vi "AddPeerNodeAtIndex.vi"(8 "error in":errorcluster, 9 "TreeIndex":i32, 10 "parent node ID":string, 11 "node in":refnum<class "NISE_CEF_Node.lvclass">) -> (0 "error out":errorcluster, 2 "summary":T1[](array[typedef]))   [LabVIEW 2015, in "Configuration Tool.lvlib"]
doc: "This Vi adds a new node to the Parent Node IDCopyright 2017 National Instruments Corporation\n\nLicensed under the Apache License, Version 2.0 (the \"License\"); you may not use this file except in compliance with the License. You may obtain a copy of the License at http://www.apache.org/licenses/LICENSE-2.0\nUnless required by applicable law or agreed to in writing, software distributed under the License is distributed on an \"AS IS\" BASIS, WITHOUT WARRANTIES OR CONDITIONS OF ANY KIND, either express or implied. See the License for the specific language governing permissions and limitations under the License."
uses:
  Configuration Tool.lvlib
  <vilib>/NI/Configuration Framework/Node/Summary.ctl
  <vilib>/NI/Configuration Framework/Node/NISE_CEF_Node.lvclass
  <vilib>/NI/Configuration Framework/Node/NISE_CEF_Node.lvclass/NISE_CEF_Node.ctl
  <vilib>/NI/Configuration Framework/Node/WriteParent.vi
  <vilib>/NI/Configuration Framework/NISE_CEF_TreeControl.lvlib
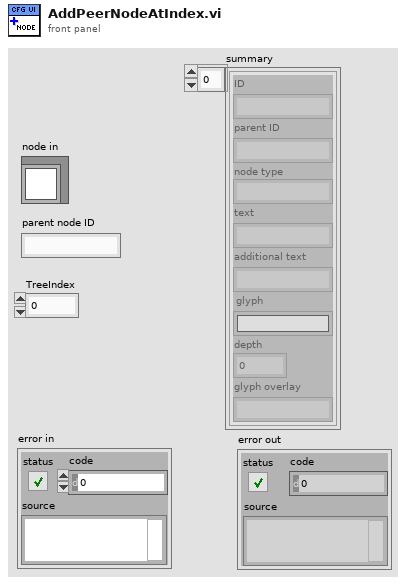
[diagram p1: front panel]
types:
  T1 = typedef "NISE_CEF_Node.lvclass/Summary.ctl" = cluster{"ID":string, "parent ID":string, "node type":string, "text":string, "additional text":string, "glyph":string, "depth":i32, "glyph overlay":string}
  T2 = typedef "NISE_CEF_Node.lvclass/NodeRef.ctl" = refnum<data-value>
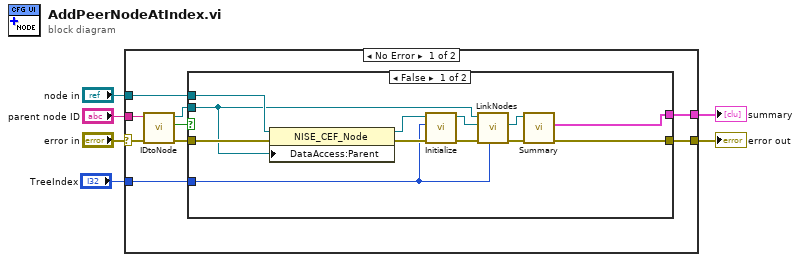
[diagram p0: block diagram]
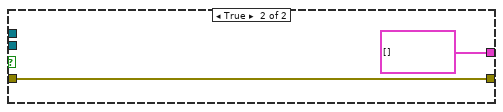
[diagram p2: hidden frame]
diagram:
  n1 = case shown="No Error" "error in" {
    selector: "error in" -> [w10 w30]
    tunnel: "parent node ID" -> [w15 _]
    tunnel: [w13 _] -> w4
    tunnel: [w12 w30] -> w3
    tunnel: "node in" -> [w11 _]
    tunnel: "TreeIndex" -> [w7 _]
    frame No Error {
      n2 = call <vilib>:"IDtoNode.vi"("error in"=w10, "ID"=w15) -> ("error out"=w9:errorcluster, "invalid Id"=w8:bool, "node ref"=w14:T2)  [unwired: 7 in]
      n3 = case shown="False" w8 {
        tunnel: w14 -> [w17 _]
        tunnel: [w27 T1[] [] ("summary")] -> w13
        tunnel: [w26 w29] -> w12
        tunnel: w11 -> [w19 _]
        tunnel: w9 -> [w21 w29]
        tunnel: w7 -> [w16 _]
        frame False {
          n4 = property class="NISE_CEF_Node"(reference=w19, error in=w21, "DataAccess:Parent"=w17) -> (reference out=w18:refnum<class "NISE_CEF_Node.lvclass">, error out=w20:errorcluster)
          n5 = call-dynamic "Initialize.vi"("error in"=w20, "parameters"=w16, "node in"=w18) -> ("error out"=w22:errorcluster, "data value reference"=w23:T2)  [unwired: 6 in, 1 out]
          n6 = call <vilib>:"LinkNodes.vi"("index"=w16, "error in"=w22, "child in"=w23, "parent in"=w17) -> ("error out"=w25:errorcluster, "child out"=w24:T2)  [unwired: 5 in, 1 out]
          n7 = call <vilib>:"Summary.vi"("error in"=w25, "node self ref"=w24) -> ("error out"=w26:errorcluster, "summary"=w27:T1[])  [unwired: 8 in]
        }
        frame True {
        }
      }
    }
    frame Error {
    }
  }
  "error out" <- w3
  "summary" <- w4
